vi "Write.vi"(8 "error in (no error)":errorcluster, 9 "channel B duty":sgl, 10 "channel A duty":sgl, 11 "Task in":refnum<class "PWM.lvclass">) -> (0 "error out":errorcluster, 3 "Task out":refnum<class "PWM.lvclass">)   [LabVIEW 2009, in "MicroDAQ.lvlib" / "PWM.lvclass"]
uses:
  <instrlib>/MicroDAQ/Channel/PWM/PWM.lvclass
  <instrlib>/MicroDAQ/Channel/PWM/PWM.lvclass/PWM.ctl
  <instrlib>/MicroDAQ/Channel/Channel.lvclass
  <instrlib>/MicroDAQ/Mlink library wraper/mlink.lvlib
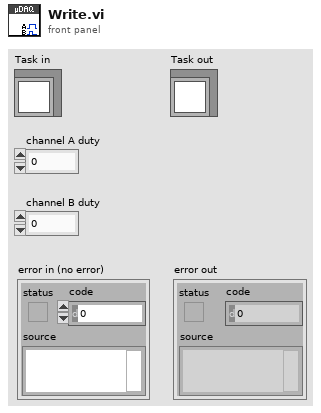
[diagram p1: front panel]
types:
  T1 = typedef "MicroDAQ.lvlib/PWM channel.ctl" = enum8{"None", "PWM1", "PWM2", "PWM3"}
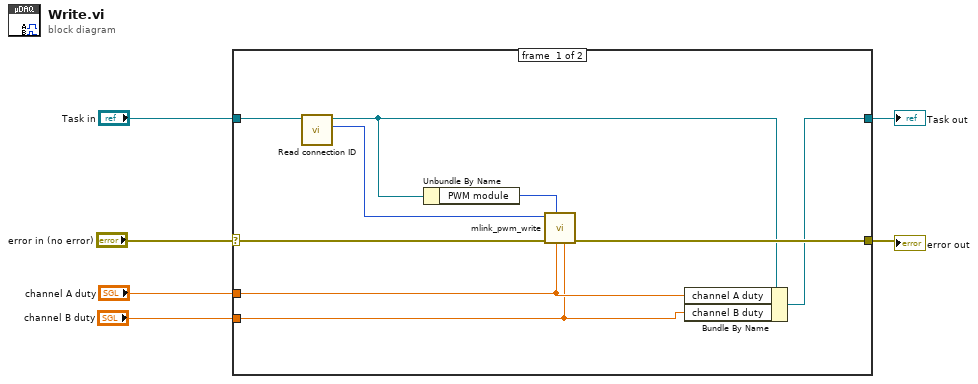
[diagram p0: block diagram]
diagram:
  n1 = case shown="No Error" "error in (no error)" {
    selector: "error in (no error)" -> [w14 w16]
    tunnel: [w13 w16] -> w5
    tunnel: "Task in" -> [w15 w17]
    tunnel: [w9 w17] -> w3
    tunnel: "channel A duty" -> [w8 _]
    tunnel: "channel B duty" -> [w7 _]
    frame #0 {
      n2 = call <instrlib>:"Read connection ID.vi"("Task in"=w15) -> ("connection ID"=w12:i32, "Task out"=w10:refnum<class "PWM.lvclass">)  [unwired: 9 in]
      n3 = Unbundle By Name(w10) -> ("PWM module"=w11:T1)
      n4 = call <instrlib>:"mlink_pwm_write.vi"("channel B"=w7, "channel A"=w8, "PWM module"=w11, "error in (no error)"=w14, "connection ID"=w12) -> ("error out"=w13:errorcluster)  [unwired: 5 in, 1 out]
      n5 = Bundle By Name(cluster=w10, "channel A duty"=w8, "channel B duty"=w7) -> (w9:refnum<class "PWM.lvclass">)
    }
    frame #1 {
    }
  }
  "error out" <- w5
  "Task out" <- w3
